vi "MTM2_salTelemetrySub_tangentActuatorPositionAbsoluteEncoderPositionMeasured.vi"(8 "error in (no error)":errorcluster) -> (0 "error out":errorcluster, 3 "function return":i32)   [LabVIEW 2018, in "SALLV_MTM2.lvlib"]
doc: "int MTM2_shm_salTelemetrySub_tangentActuatorPositionAbsoluteEncoderPositionMeasuredLV();"
uses:
  SALLV_MTM2.lvlib
  SALLV_MTM2.so
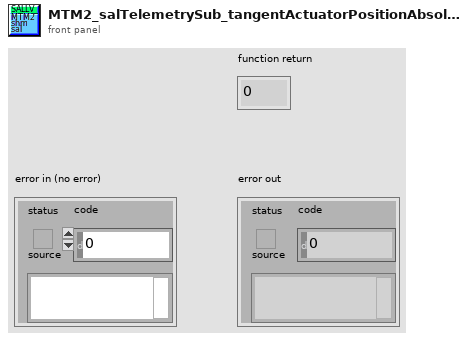
[diagram p1: front panel]
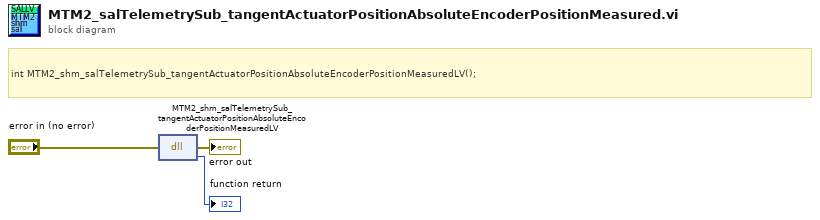
[diagram p0: block diagram]
diagram:
  # "int MTM2_shm_salTelemetrySub_tangentActuatorPositionAbsoluteEncoderPositionMeasuredLV();"
  n1 = dll-call lib="home/ttsai/Document/salApiMTM2/SALLV_MTM2/SALLV_MTM2.*" fn="MTM2_shm_salTelemetrySub_tangentActuatorPositionAbsoluteEncoderPositionMeasuredLV"(error in="error in (no error)") -> (error out=→"error out":errorcluster, →"function return":i32)  [unwired: 2 in, 1 out]
